vi "RTM - Remove Channels Dependency.vi"(8 "error in (no error)":errorcluster, 9 "Menu hierarchy in":string[](array[string]), 11 "Node Ptr":u64 format="%.0x") -> (0 "error out":errorcluster, 1 "Menu hierarchy out":string[](array[string]), 3 "Action":T1)   [LabVIEW 2016, in "UDP-Custom-Device System Explorer.lvlib"]
uses:
  UDP-Custom-Device System Explorer.lvlib
  <vilib>/NI Veristand/Custom Device API/Custom Device RTM Dependency.ctl
  <vilib>/NI VeriStand/Custom Device API/Custom Device API.lvlib
  Property Accessors/Shared Packet Accessors.lvlib
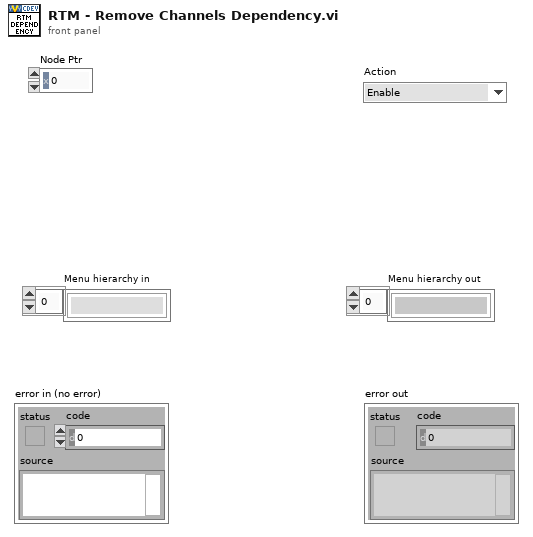
[diagram p1: front panel]
types:
  T1 = typedef "Custom Device API.lvlib/Custom Device RTM Dependency.ctl" = enum16{"Enable", "Disable", "Hide"}
  T2 = typedef "Custom Device API.lvlib/Custom Device Item Ref.ctl" = u64
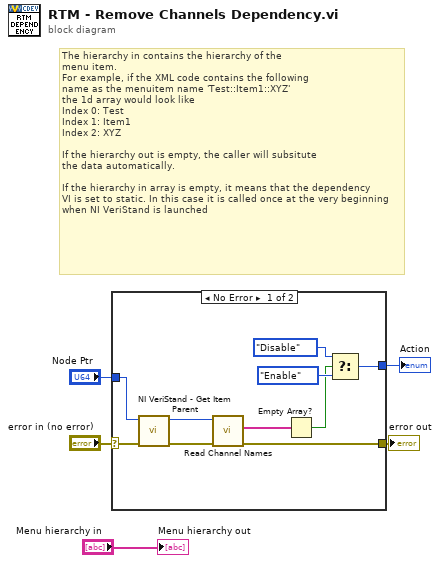
[diagram p0: block diagram]
diagram:
  # "The hierarchy in contains the hierarchy of the\nmenu item.\nFor example, if the XML code contains the following\nname as the menuitem name 'Test::Item1::XYZ'\nthe 1d array would look like\nIndex 0: Test\nIndex 1: Item1\nIndex 2: XYZ\n\nIf the hierarchy out is empty, the caller will subsitute\nthe data automatically.\n\nIf the hierarchy in array is empty, it means that the dependency\nVI is set to static. In this case it is called once at the very beginning\nwhen NI VeriStand is launched"
  n1 = case shown="No Error" "error in (no error)" {
    selector: "error in (no error)" -> [w11 w16]
    tunnel: "Node Ptr" -> [w10 _]
    tunnel: [w15 _] -> w3
    tunnel: [w7 w16] -> w1
    frame No Error {
      n2 = call <vilib>:"NI VeriStand - Get Item Parent.vi"("error in (no error)"=w11, "Item Ref in"=w10) -> ("error out"=w6:errorcluster, "Item Ref out"=w9:T2)  [unwired: 6 in, 2 out]
      n3 = call "Read Channel Names.vi"("error in (no error)"=w6, "Node Ptr"=w9) -> ("error out"=w7:errorcluster, "Channel Names"=w8:string[])  [unwired: 7 in, 1 out]
      n4 = Empty Array?(array=w8) -> (empty?=w12:bool)
      n5 = Select(t=Custom_Device_RTM_Dependency."Disable" ("Action"), s=w12, f=Custom_Device_RTM_Dependency."Enable" ("Action")) -> (s? t:f=w15:T1)
    }
    frame Error {
    }
  }
  "error out" <- w1
  "Action" <- w3
  "Menu hierarchy out" <- "Menu hierarchy in"
